vi "Test osk.vi"() -> ()   [LabVIEW 2012]
panel:
  in  "String":string
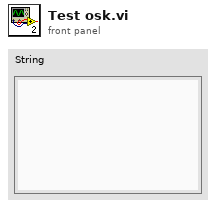
[diagram p1: front panel]
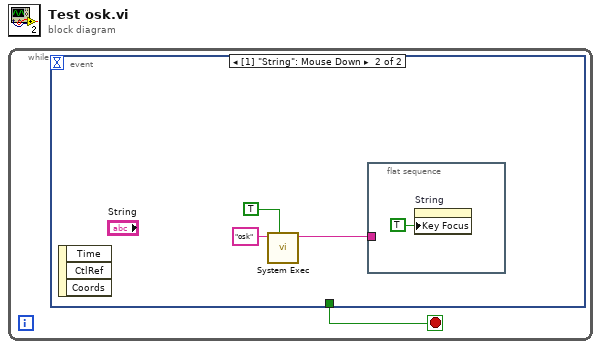
[diagram p0: block diagram]
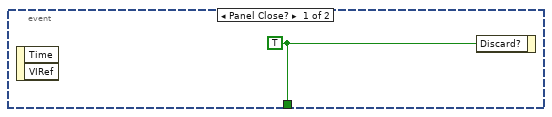
[diagram p2: hidden frame]
diagram:
  n1 = while {
    stop <- w1 stop-if-true
    n2 = event shown="[1] \"String\": Mouse Down" {
      selector: _ -> [_ _]
      dyn-events: _ -> [_ _]
      timeout: _ -> [_ _]
      tunnel: [w2 _] -> w1
      event Panel Close? {
        w2 = TRUE ("Discard?")
        n3 = event-data() -> ()  [unwired: 1 in, 2 out]
        n4 = event-data("Discard?"=w2) -> ()  [unwired: 1 in, 1 out]
      }
      event "String": Mouse Down {
        n5 = event-data() -> ()  [unwired: 1 in, 3 out]
        n6 = call <vilib>:"System Exec.vi"("wait until completion? (T)"=TRUE, "command line"="osk") -> ("standard output"=w3:string)  [unwired: 6 in, 3 out]
        n7 = flat-sequence {
          tunnel: w3 -> [_]
          frame #0 {
            n8 = property on="String" class="Str"("Key Focus"=TRUE) -> ()  [unwired: 2 in, 2 out]
          }
        }
      }
    }
  }
